vi "find conflict mode.vi"() -> ()   [LabVIEW 2019]
uses:
  Stand_class/Valve Mode.ctl
  c5223ed3-29bc-43e4-bc30-907d8cbfd681.vi
  b00310a7-8dd4-48a1-b87f-47ca66113c7f.vi
  58279113-44f2-4d30-ba2a-0af0d3c2a27b.vi
  Stand_class/Valve State Mode.vi/810e184e-eeb6-4027-a8ae-1422f3ce3d45.vi
  Stand_class/Valve State Mode.vi/57bd4a65-f3dc-44f5-8d68-677c2a197570.vi
  Stand_class/Valve State Mode.vi/03b2f9e4-fceb-4725-9b90-3fd10082a088.vi
  Stand_class/Valve State Mode.vi/3d0d09bd-48e8-482f-b1e2-a36b2bb65234.vi
  Stand_class/Valve State Mode.vi/33d3f26a-dc4a-4f56-bf0a-61d04c5d7434.vi
  Stand_class/Valve State Mode.vi/52af9d47-24d1-4057-80bf-8d93bfb3d17d.vi
  Stand_class/Valve State Mode.vi/094228cb-a119-423c-9af8-5a16f059a318.vi
  Stand_class/Valve State Mode.vi/bf5ad1e6-a0ae-4579-ad74-ca8f304cb7cf.vi
  Stand_class/Valve State Mode.vi/eb4d2b76-f0f0-4e1d-bda0-609c5f37b4e7.vi
  Stand_class/Const All Valve.vi
panel:
  in  "Array":T1[](array[typedef])=[enum."Pump Pressure DUT", enum."Pump Pressure Chamber", enum."Haskel Pressure DUT", enum."Haskel Pressure Chamber", enum."Slow Release DUT", enum."Slow Release Chamber", enum."Fast Release DUT", enum."Fast Release Chamber", enum."Fast Release DUT and Chamber", enum."Leak Pressure DUT", enum."Leak Pressure Chamber", enum."Back Pressure DUT", enum."Back Pressure Chamber"]
  out "Set":set{set{T1}}(c389)
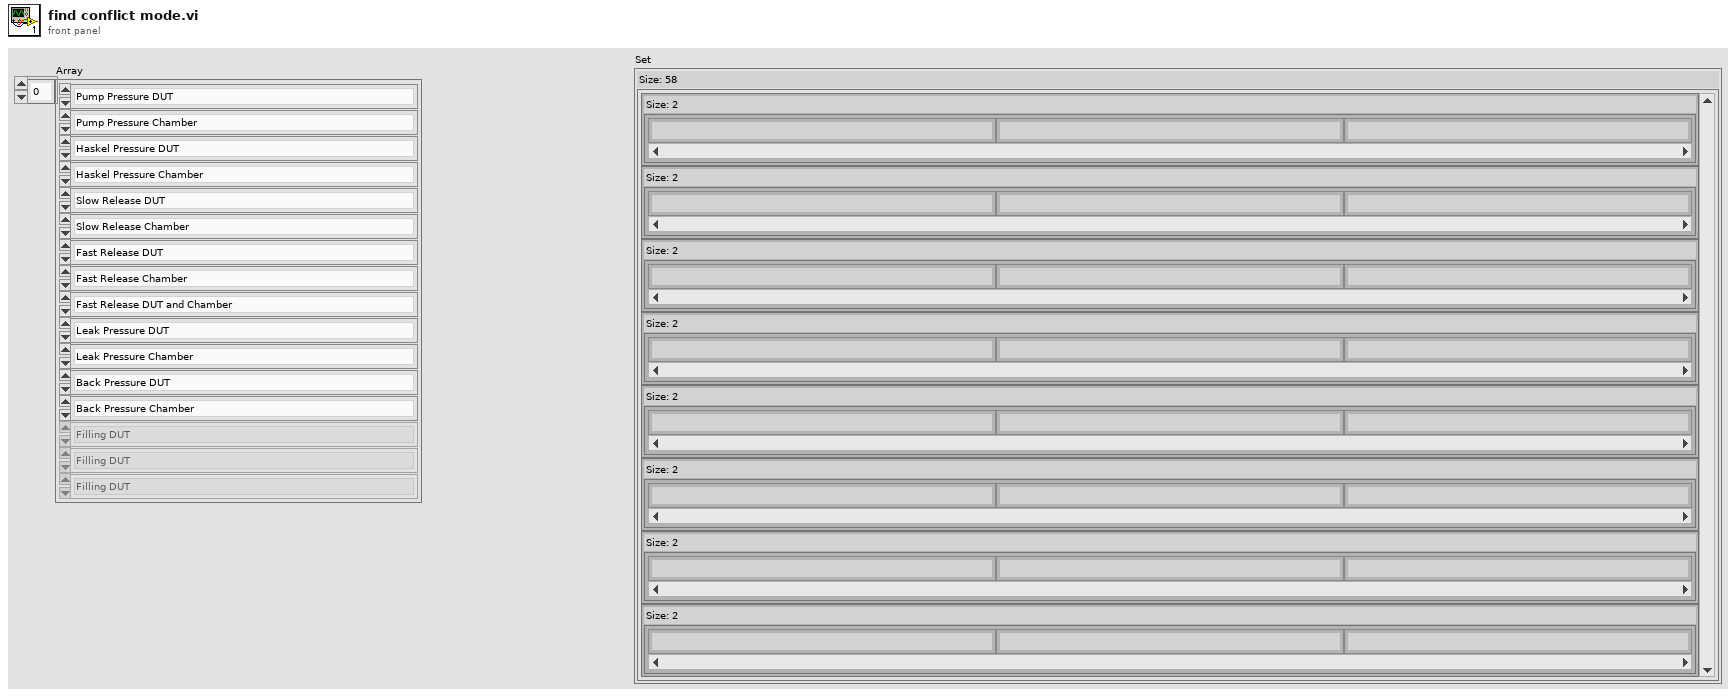
[diagram p1: front panel]
types:
  T1 = typedef "Valve Mode.ctl" = enum16{"Filling DUT", "Filling Chamber", "Pump Pressure DUT", "Pump Pressure Chamber", "Haskel Pressure DUT", "Haskel Pressure Chamber", "Slow Release DUT", "Slow Release Chamber", "Fast Release DUT", "Fast Release Chamber", "Fast Release DUT and Chamber", "Leak Pressure DUT", "Leak Pressure Chamber", "Back Pressure DUT", "Back Pressure Chamber", "Fully Closed"}
  T2 = typedef "DO index.ctl" = u8
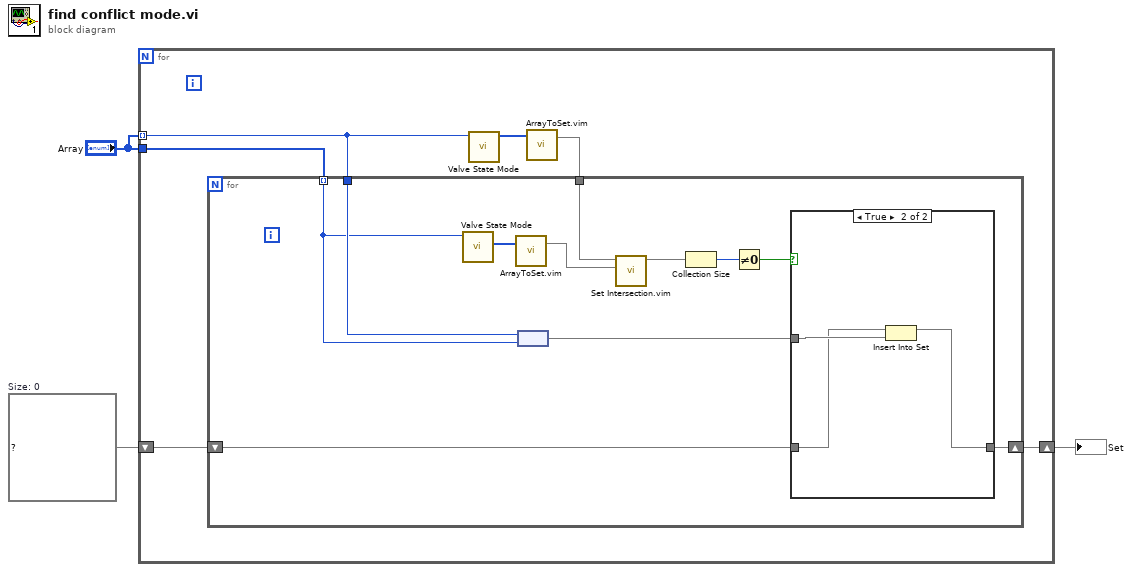
[diagram p0: block diagram]
diagram:
  w3 = set{set{T1}} {}  # Size: 0
  n1 = for {
    shift-right: [w7] -> w2
    shift-left: w3 -> [w6]
    tunnel: "Array" -> [w5] mode=indexing
    tunnel: "Array" -> [w4]
    n2 = call "Valve State Mode.vi"("Valve Mode"=w5) -> ("open"=w9:T2[])  [unwired: 9 in, 1 out]
    n3 = call "ArrayToSet.vim"("Array"=w9) -> ("Set"=w8:set{T2})  [unwired: 2 in]
    n4 = for {
      tunnel: w8 -> [w19]
      tunnel: w5 -> [w15]
      shift-right: [w12] -> w7
      shift-left: w6 -> [w11]
      tunnel: w4 -> [w10] mode=indexing
      n5 = call "Valve State Mode.vi"("Valve Mode"=w10) -> ("close"=w20:T2[])  [unwired: 9 in, 1 out]
      n6 = call "ArrayToSet.vim"("Array"=w20) -> ("Set"=w18:set{T2})  [unwired: 2 in]
      n7 = node(w15, w10) -> (w13:set{T1})
      n8 = call "Set Intersection.vim"("set 2"=w18, "set 1"=w19) -> ("intersection"=w17:set{T2})  [unwired: 9 in]
      n9 = Collection Size(1:w17) -> (0:w16:i32)
      n10 = Not Equal To 0?(x=w16) -> (x != 0?=w14:bool)
      n11 = case shown="True" w14 {
        tunnel: w13 -> [_ w24]
        tunnel: [w21 w23] -> w12
        tunnel: w11 -> [w21 w22]
        frame False {
        }
        frame True {
          n12 = Insert Into Set(10:w24, 11:w22) -> (3:w23:set{set{T1}})  [unwired: 1 out]
        }
      }
    }
  }
  "Set" <- w2
